vi "Funktionen Schalten - Dichtheitstest.vi"() -> (2 "Ventile Dichtheitstest":T1)   [LabVIEW 2020, in "Allgemein.lvlib"]
uses:
  Allgemein.lvlib
  Konfig-Dateien/FGV Betriebsdaten Aktionen.ctl
  Konfig-Dateien/Konfig-Dateien.lvlib
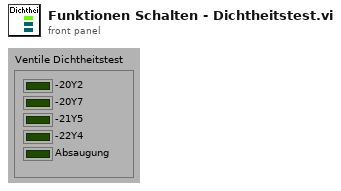
[diagram p1: front panel]
types:
  T1 = cluster{"-20Y2":bool, "-20Y7":bool, "-21Y5":bool, "-22Y4":bool, "Absaugung":bool}
  T2 = typedef "Konfig-Dateien.lvlib/FGV Betriebsdaten Aktionen.ctl" = enum16{"lesen", "Anlagengrenzw.", "PID Param.", "Sonstige", "Sensor Para."}
  T3 = typedef "Erweiterte Konfig.lvlib/Sonstige Parameter.ctl" = cluster{"Lüfter langsam":sgl, "Lüfter schnell":sgl, "FT-IR Kühlung Soll":sgl, "FT-IR Kühlung Max":sgl, "Überwachung":T4, "Befüllung aktiv":T5, "Stickstoff Befüllzeit":sgl, "Befüllintervall":sgl, "Kalibrierwert FT-IR":sgl, "Offset Ausgang":sgl, "Offset FT-IR":sgl, "Offset Druck FT-IR":sgl, "Dichtheitstest Zeit":sgl, "Dichtheitstest Abfall":sgl, "Dichtheitstest Umfang":T6, "Offset Umgebung":sgl, "Max Taupunkt":sgl, "Pumpendrehzahl":sgl}
  T4 = typedef "Auswahlfeld.ctl" = u16
  T5 = typedef "LogKonfig.lvlib/Auswahlfeld aktiviert-deaktiviert.ctl" = u16
  T6 = typedef "Erweiterte Konfig.lvlib/Dichtheitstest Umfang.ctl" = u16
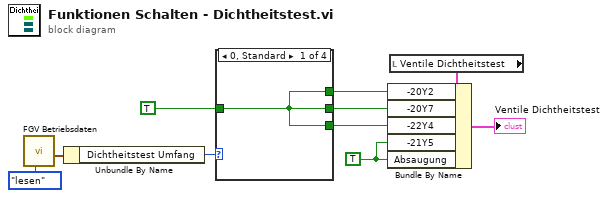
[diagram p0: block diagram]
diagram:
  w3 = TRUE
  n1 = call "FGV Betriebsdaten.vi"("Aktionen"=FGV_Betriebsdaten_Aktionen."lesen") -> ("Sonstige"=w4:T3)  [unwired: 7 in, 3 out]
  n2 = Unbundle By Name(w4) -> ("Dichtheitstest Umfang"=w10:T6)
  n3 = case shown="0, Standard" w10 {
    tunnel: TRUE -> [w11 w12 w13 _]
    tunnel: [w11 w12 _ _] -> w2
    tunnel: [w11 _ _ _] -> w6
    tunnel: [w11 w12 w13 _] -> w1
    frame 0, Default {
    }
    frame 1 {
    }
    frame 2 {
    }
    frame 3 {
    }
  }
  n4 = local read "Ventile Dichtheitstest"() -> (w8:T1)
  n5 = Bundle By Name(cluster=w8, "-20Y2"=w2, "-20Y7"=w1, "-22Y4"=w6, "-21Y5"=w3, "Absaugung"=w3) -> (→"Ventile Dichtheitstest":T1)
